vi "Conversion Constants.vi"() -> ()   [LabVIEW 2016]
panel:
  in  "psi to mb":dbl=68.9475729
  in  "mb to Pa":dbl=100.0
  in  "lpm to m3/s":dbl=1.6666666666666667e-05
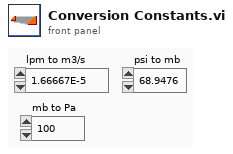
[diagram p1: front panel]
diagram:
